vi "RoboControl7.vi"   [LabVIEW 2015]
uses:
  GlobalVISA7.vi
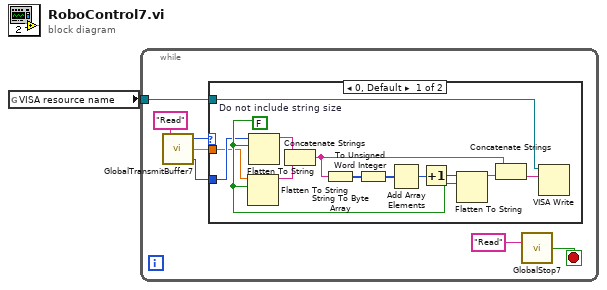
[diagram p0: block diagram]
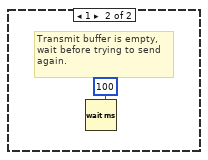
[diagram p2: hidden frame]
diagram:
  n1 = global read "GlobalVISA7.vi" "VISA resource name"() -> (w1:refnum<visa-resource-name>)
  n2 = while {
    tunnel: w1 -> [w2]
    stop <- w7 stop-if-true
    n3 = call "GlobalTransmitBuffer7.vi"("Function select"="Read") -> ("Data_ID # out"=w3:u16, "Value out"=w4:sgl, "Result status\n(0 = success)"=w5:i32)  [unwired: 2 in]
    n4 = case shown="0, Default" w5 {
      tunnel: w4 -> [w10 _]
      tunnel: w3 -> [w11 _]
      tunnel: w2 -> [w13 _]
      frame 0, Default {
        w12 = FALSE  # Do not include string size
        n5 = Flatten To String(anything=w10, prepend array or string size? (T)=w12) -> (data string=w20:string)  [unwired: 2 in, 2 out]
        n6 = Flatten To String(anything=w11, prepend array or string size? (T)=w12) -> (data string=w21:string)  [unwired: 2 in, 2 out]
        n7 = Concatenate Strings(w21, w20) -> (w14:string)
        n8 = String To Byte Array(string=w14) -> (unsigned byte array=w19:u8[])
        n9 = To Unsigned Word Integer(number=w19) -> (unsigned 16bit integer=w18:u16[])
        n10 = Add Array Elements(numeric array=w18) -> (sum=w17:u16)
        n11 = Increment(x=w17) -> (x+1=w16:u16)
        n12 = Flatten To String(anything=w16, prepend array or string size? (T)=w12) -> (data string=w15:string)  [unwired: 2 in, 2 out]
        n13 = Concatenate Strings(w14, w15) -> (w9:string)
        n14 = VISA Write(VISA resource name=w13, write buffer=w9) -> ()  [unwired: 1 in, 3 out]
      }
      frame 1 {
        # "Transmit buffer is empty,\nwait before trying to send\nagain."
        n15 = Wait (ms)(milliseconds to wait=100) -> ()  [unwired: 1 out]
      }
    }
    n16 = call "GlobalStop7.vi"("Function select"="Read") -> ("stop"=w7:bool)
  }
